vi "DecToNin.vi"(11 "Decimal":dbl) -> (0 "10^x":string, 1 "Nin":string, 2 "10^x":dbl, 3 "N in":dbl)   [LabVIEW 2017]
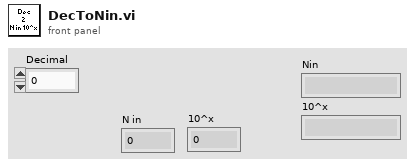
[diagram p1: front panel]
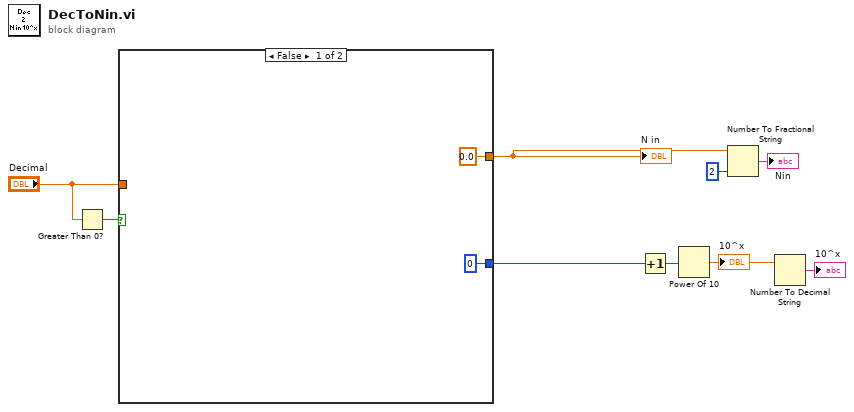
[diagram p0: block diagram]
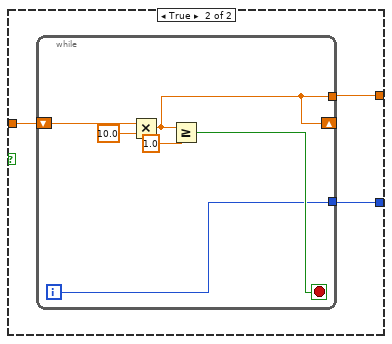
[diagram p2: hidden frame]
diagram:
  n1 = Greater Than 0?(x="Decimal") -> (x > 0?=w1:bool)
  n2 = case shown="False" w1 {
    tunnel: "Decimal" -> [_ w14]
    tunnel: [0 w13] -> w9
    tunnel: [0.0 w12] -> w7
    frame False {
    }
    frame True {
      n3 = while {
        tunnel: [w16] -> w13
        tunnel: [w15] -> w12
        shift-right: [w15] -> _
        shift-left: w14 -> [w20]
        i -> [w16]
        stop <- w17 stop-if-true
        n4 = Multiply(x=w20, y=10.0) -> (x*y=w15:dbl)
        n5 = Greater Or Equal?(x=w15, y=1.0) -> (x >= y?=w17:bool)
      }
    }
  }
  "N in" <- w7
  n6 = Increment(x=w9) -> (x+1=w8:i32)
  n7 = Power Of 10(x=w8) -> (10^x=w4:dbl)
  "10^x" <- w4
  n8 = Number To Fractional String(number=w7, precision (6)=i16 2) -> (F-format string=→"Nin":string)  [unwired: 2 in]
  n9 = Number To Decimal String(number=w4) -> (decimal integer string=→"10^x":string)  [unwired: 1 in]
